vi "Largest Contiguous Channel Count.vi"   [LabVIEW 2017, in "DSF Core.lvlib"]
uses:
  DSF Core.lvlib
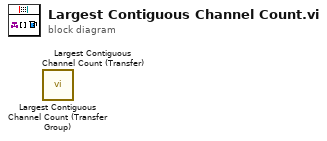
[diagram p0: block diagram]
diagram:
  n1 = call "Largest Contiguous Channel Count (Transfer Group).vi"() -> ()  [unwired: 9 in, 3 out]
  n2 = call "Largest Contiguous Channel Count (Transfer).vi"() -> ()  [unwired: 9 in, 3 out]
